vi "UnescapeWhitespace.vi"(10 "EscapedWhitespace":string) -> (2 "OutputString":string)   [LabVIEW 2022 SP3, in "StringUtils.lvlib"]
uses:
  StringUtils.lvlib
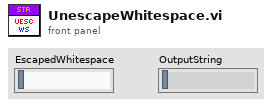
[diagram p1: front panel]
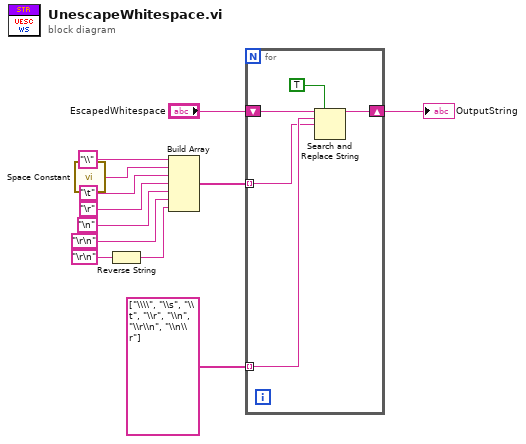
[diagram p0: block diagram]
diagram:
  n1 = call <vilib>:"Space Constant.vi"() -> ("String"=w12:string)
  n2 = Reverse String(1:"\r\n") -> (0:w6:string)
  n3 = Build Array("\\", w12, "\t", "\r", "\n", "\r\n", w6) -> (w1:string[])
  n4 = for {
    shift-right: [w16] -> w3
    shift-left: "EscapedWhitespace" -> [w17]
    tunnel: w1 -> [w13] mode=indexing
    tunnel: string[] ["\\\\", "\\s", "\\t", "\\r", "\\n", "\\r\\n", "\\n\\r"] -> [w14] mode=indexing
    n5 = Search and Replace String(replace all?=TRUE ("replace all? (F)"), input string=w17, search string=w14, replace string=w13) -> (result string=w16:string)  [unwired: 4 in, 3 out]
  }
  "OutputString" <- w3
